vi "communicateReplacementErForceSimulator.vi"(4 "replaceRobots":bool, 5 "degubBall":bool=TRUE, 6 "Game":refnum<class "Game.lvclass">, 7 "replaceBall":bool=TRUE, 8 "error in (no error)":errorcluster, 9 "grSIM replacement":T1, 10 "Com UDP":T4={"UDP GrSim TX"=TRUE, "Address:"="172.17.88.61", "Port:"=10301}, 11 "Communication in":refnum<class "Communication.lvclass">) -> (0 "error out":errorcluster, 3 "Communication out":refnum<class "Communication.lvclass">)   [LabVIEW 2020, in "Communication.lvclass"]
uses:
  Communication.lvclass
  Controls/ComUDP.ctl
  Controls/grSimReplacement.ctl
  Paths/grSim Packet Command UDP Test Folder/grSim/grSim RobotReplacement.ctl
  Paths/grSim Packet Command UDP Test Folder/grSim/grSim_BallReplacement.ctl
  Game_class/Game.lvclass
  Game_class/Game.lvclass/Game.ctl
  Game_class/Read BallRef.vi
  Ball_class/Ball.lvclass
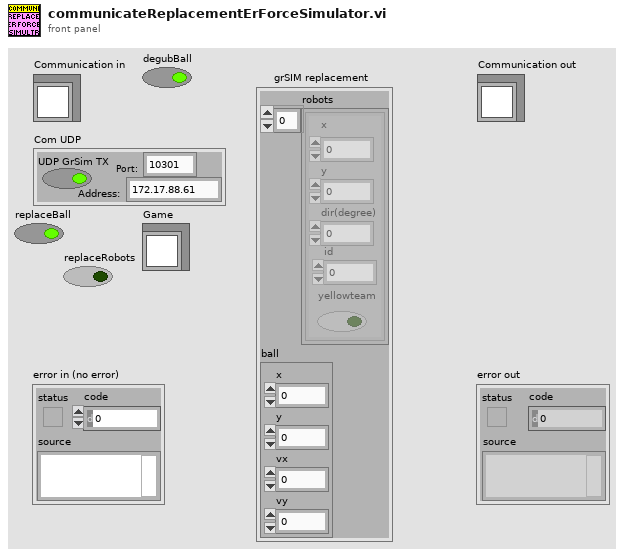
[diagram p1: front panel]
types:
  T1 = typedef "grSimReplacement.ctl" = cluster{"robots":T2[], "ball":T3}
  T2 = typedef "grSim RobotReplacement.ctl" = cluster{"x":dbl, "y":dbl, "dir(degree)":dbl, "yellowteam":bool, "id":u32}
  T3 = typedef "grSim_BallReplacement.ctl" = cluster{"x":dbl, "y":dbl, "vx":dbl, "vy":dbl}
  T4 = typedef "ComUDP.ctl" = cluster{"UDP GrSim TX":bool, "Address:":string, "Port:":u16}
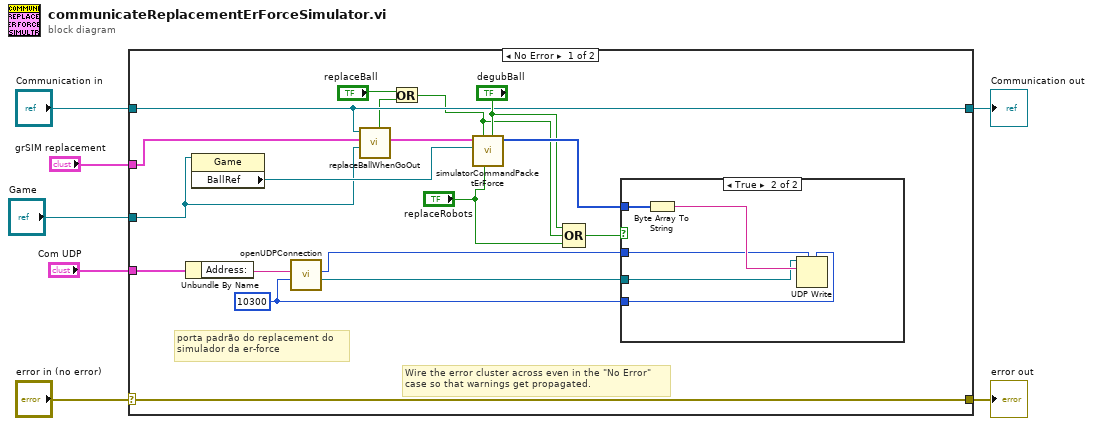
[diagram p0: block diagram]
diagram:
  n1 = case shown="No Error" "error in (no error)" {
    selector: "error in (no error)" -> [w25 w32]
    tunnel: [w25 w32] -> w6
    tunnel: [w11 w31] -> w4
    tunnel: "Communication in" -> [w11 w31]
    tunnel: "Com UDP" -> [w24 _]
    tunnel: "grSIM replacement" -> [w14 _]
    tunnel: "Game" -> [w12 _]
    frame No Error {
      w20 = u16 10300 ("Port:")
      # "porta padrão do replacement do\nsimulador da er-force"
      # "Wire the error cluster across even in the \"No Error\"\ncase so that warnings get propagated."
      n2 = Unbundle By Name(w24) -> ("Address:"=w23:string)
      n3 = property class="Game"(reference=w12) -> ("BallRef"=w15:refnum<class "Ball.lvclass">)  [unwired: 1 in, 2 out]
      n4 = call "openUDPConnection.vi"("Port:"=w20, "SSL Vision Address:"=w23) -> ("connectionID out"=w22:refnum<k16>, "IP Address"=w21:u32)  [unwired: 6 in, 2 out]
      n5 = call "replaceBallWhenGoOut.vi"("Game"=w12, "grSIM replacement"=w14, "Communication in"=w11) -> ("grSIM replacement out"=w13:T1, "replaceBall"=w8:bool)  [unwired: 5 in, 2 out]
      n6 = Or(x="replaceBall", y=w8) -> (x .or. y?=w9:bool)
      n7 = call "simulatorCommandPacketErForce.vi"("degubBall"="degubBall", "replaceRobots"="replaceRobots", "replaceBall"=w9, "Ball"=w15, "grSIM replacement"=w13) -> ("Array"=w19:u8[])  [unwired: 6 in]
      n8 = Compound Arithmetic op=OR("degubBall", w9, "replaceRobots") -> (w18:bool)
      n9 = case shown="True" w18 {
        tunnel: w22 -> [_ w29]
        tunnel: w21 -> [_ w28]
        tunnel: w20 -> [_ w27]
        tunnel: w19 -> [_ w26]
        frame False {
        }
        frame True {
          n10 = Byte Array To String(unsigned byte array=w26) -> (string=w30:string)
          n11 = UDP Write(address=w28, port or service name=w27, connection ID=w29, data in=w30) -> ()  [unwired: 2 in, 2 out]
        }
      }
    }
    frame Error {
    }
  }
  "error out" <- w6
  "Communication out" <- w4
